vi "Ex5strip5GraphNI.vi"() -> ()   [LabVIEW 2010]
panel:
  in  "Flip":bool
  in  "Reverse":bool=TRUE
  in  "Intensifier Mode":enum16{"Safe", "Shutter", "Gate"}(ring)
  in  "IntensifierGain":u32=100
  out "Segment 5":T1(graph)
  out "Segment 4":T1(graph)
  out "Segment 3":T1(graph)
  out "Segment 2":T1(graph)
  out "Segment 1":T1(graph)
  in  "Calibration ini":path
  in  "ROI 5 Y2":u32=240
  in  "ROI 5 Y1":u32=208
  in  "ROI 4 Y2":u32=192
  in  "ROI 4 Y1":u32=160
  in  "ROI 3 Y2":u32=144
  in  "ROI 3 Y1":u32=112
  in  "ROI 2 Y2":u32=96
  in  "ROI 2 Y1":u32=64
  in  "ROI 1 Y2":u32=48
  in  "ROI 1 Y1":u32=16
  in  "Temperature":dbl=-10.0 format="%.2f"
  in  "Exposure":dbl=0.1 min=0.0 step=0.001 format="%.3f"
  in  "stop":bool
  out "error out":errorcluster
  in  "error in (no error)":errorcluster
  # "Calibration ini file"
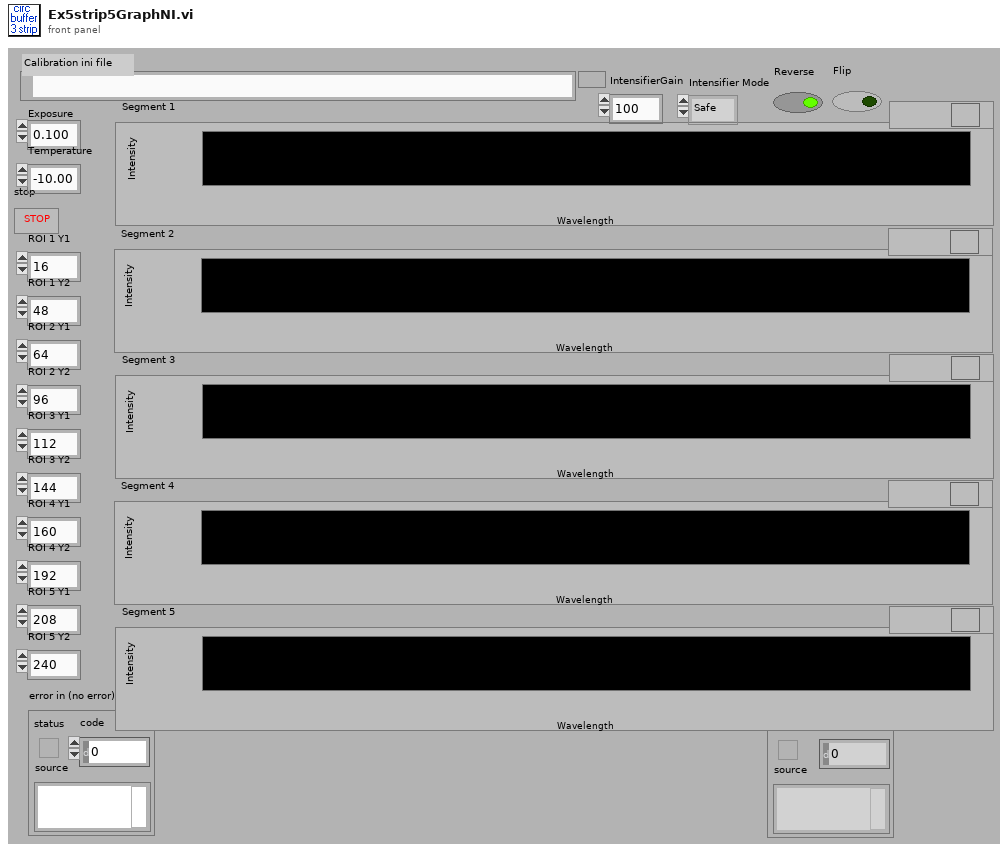
[diagram p1: front panel]
types:
  T1 = cluster{"Calibrated Array":dbl[], "Array F32":sgl[]}
  T2 = cluster{"ROI 1 Y1":u32, "ROI 1 Y2":u32, "ROI 2 Y1":u32, "ROI 2 Y2":u32, "ROI 3 Y1":u32, "ROI 3 Y2":u32, "ROI 4 Y1":u32, "ROI 4 Y2":u32, "ROI 5 Y1":u32, "ROI 5 Y2":u32}
  T3 = cluster{"Acquire focus mode,\nSync (circualar buffers)":i32, "Exposure":dbl, "Number of Images":i32, "Software Accumulation":i32}
  T4 = cluster{"Camera Handle":u32, "Pulser Handle":u32, "File Handle":u32, "Display Handle":u32, "Image Handle":u32}
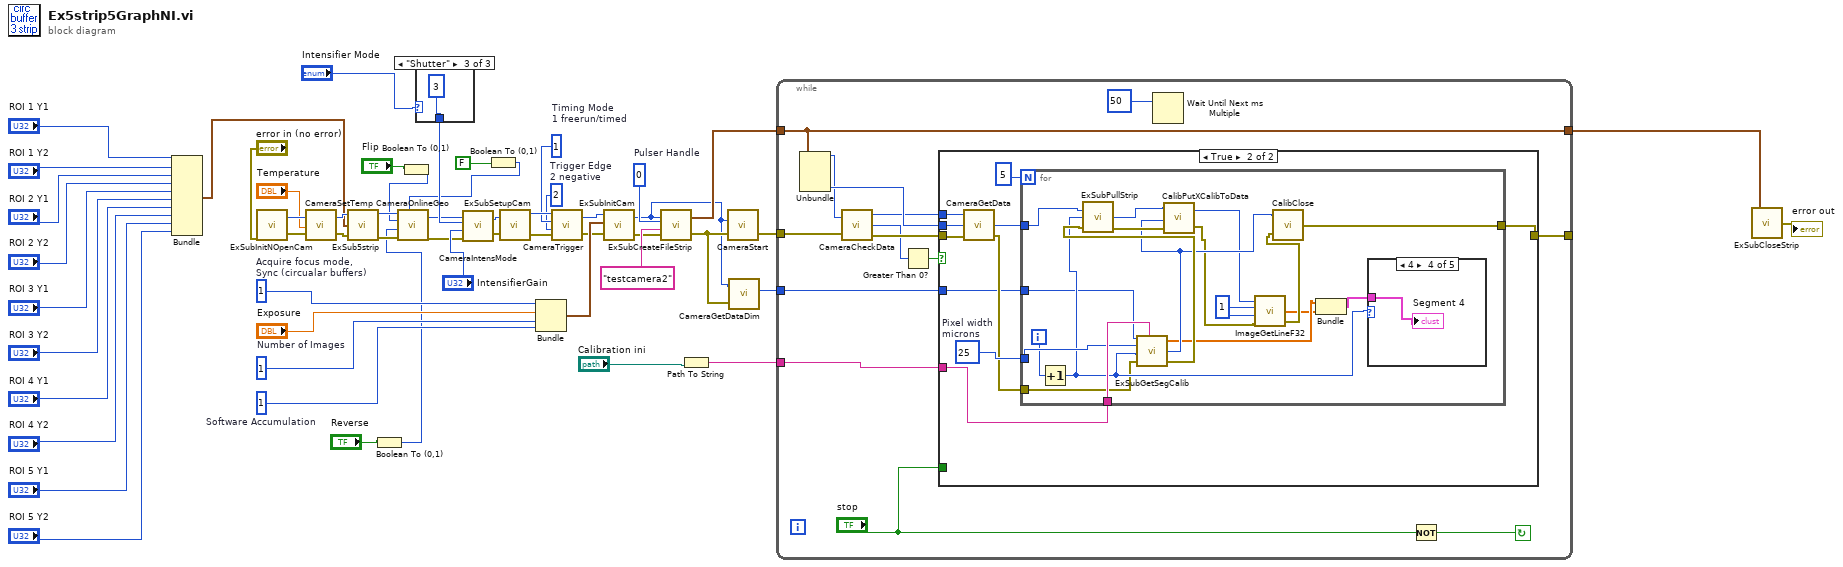
[diagram p0: block diagram]
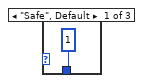
[diagram p2: hidden frame]
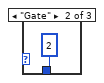
[diagram p3: hidden frame]
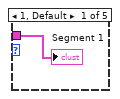
[diagram p5: hidden frame]
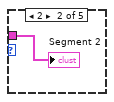
[diagram p6: hidden frame]
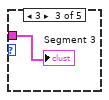
[diagram p7: hidden frame]
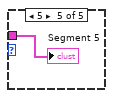
[diagram p8: hidden frame]
diagram:
  w39 = 2  # Trigger Edge 2 negative
  w40 = 1  # Timing Mode 1 freerun/timed
  w47 = 0  # Pulser Handle
  w53 = 1  # Number of Images
  w54 = 1  # Acquire focus mode, Sync (circualar buffers)
  w52 = 1  # Software Accumulation
  n1 = Bundle("ROI 1 Y1"="ROI 1 Y1", "ROI 1 Y2"="ROI 1 Y2", "ROI 2 Y1"="ROI 2 Y1", "ROI 2 Y2"="ROI 2 Y2", "ROI 3 Y1"="ROI 3 Y1", "ROI 3 Y2"="ROI 3 Y2", "ROI 4 Y1"="ROI 4 Y1", "ROI 4 Y2"="ROI 4 Y2", "ROI 5 Y1"="ROI 5 Y1", "ROI 5 Y2"="ROI 5 Y2") -> (w21:T2)  [unwired: 1 in]
  n2 = call "ExSubInitNOpenCam.vi"("error in (no error)"="error in (no error)") -> ("Camera Handle"=w34:u32, "error out"=w35:errorcluster)
  n3 = call <userlib>:"CameraSetTemp.vi"("error in (no error)"=w35, "Temperature"="Temperature", "Camera Handle"=w34) -> ("error out"=w36:errorcluster, "Camera Handle"=w33:u32)
  n4 = call "ExSub5strip.vi"("error in (no error)"=w36, "5 ROIS"=w21, "Camera Handle"=w33) -> ("error out"=w8:errorcluster, "Camera Handle"=w7:u32)
  n5 = Boolean To (0,1)(Boolean="Reverse") -> (0, 1=w3:i16)
  n6 = Boolean To (0,1)(Boolean="Flip") -> (0, 1=w5:i16)
  n7 = case shown="\"Shutter\"" "Intensifier Mode" {
    tunnel: [1 2 3] -> w15
    frame "Safe", Default {
    }
    frame "Gate" {
    }
    frame "Shutter" {
    }
  }
  n8 = Boolean To (0,1)(Boolean=FALSE) -> (0, 1=w1:i16)
  n9 = call <userlib>:"CameraOnlineGeo.vi"("Camera Handle"=w7, "Flip Flag"=w5, "Reverse Flag"=w3, "error in"=w8, "Rotate Flag"=w1) -> ("Camera Handle"=w10:u32, "error out"=w9:errorcluster)
  n10 = call <userlib>:"CameraIntensMode.vi"("error in"=w9, "Intensifier Gain"="IntensifierGain", "Mode"=w15, "Camera Handle"=w10) -> ("error out"=w14:errorcluster, "Camera Handle"=w13:u32)
  n11 = call "ExSubSetupCam.vi"("error in (no error)"=w14, "Camera Handle"=w13) -> ("error out"=w38:errorcluster, "Camera Handle"=w42:u32)
  n12 = Bundle("Acquire focus mode,\nSync (circualar buffers)"=w54, "Exposure"="Exposure", "Number of Images"=w53, "Software Accumulation"=w52) -> (w49:T3)  [unwired: 1 in]
  n13 = call <userlib>:"CameraTrigger.vi"("error in"=w38, "Trigger Edge"=w39, "Timing Mode"=w40, "Camera Handle"=w42) -> ("error out"=w43:errorcluster, "Camera Handle"=w41:u32)
  n14 = call "ExSubInitCam.vi"("error in (no error)"=w43, "Camera Information"=w49, "Camera Handle"=w41) -> ("error out"=w48:errorcluster, "Camera Handle"=w17:u32)
  n15 = call "ExSubCreateFileStrip.vi"("error in (no error)"=w48, "File and Display Name"="testcamera2", "Pulser Handle"=w47, "Camera Handle"=w17) -> ("error out"=w18:errorcluster, "Handles Out"=w46:T4)
  n16 = Path To String(path="Calibration ini") -> (string=w19:string)
  n17 = call <userlib>:"CameraStart.vi"("error in"=w18, "Camera Handle"=w17) -> ("error out"=w37:errorcluster)  [unwired: 1 out]
  n18 = call <userlib>:"CameraGetDataDim.vi"("Camera Handle"=w17, "error in"=w18) -> ("Xdim"=w16:u32)  [unwired: 3 out]
  n19 = while {
    tunnel: w46 -> [w70]
    tunnel: w37 -> [w69]
    tunnel: [w67] -> _
    tunnel: [w70] -> w45
    tunnel: w19 -> [w61]
    tunnel: w16 -> [w59]
    stop <- w71 continue-if-true
    n20 = Unbundle(w70) -> ("Camera Handle"=w65:u32, "Image Handle"=w66:u32)  [unwired: 3 out]
    n21 = call <userlib>:"CameraCheckData.vi"("Camera Handle"=w65, "error in"=w69) -> ("Camera Handle"=w64:u32, "Number Of Frames Available"=w62:i32, "error out"=w68:errorcluster)
    n22 = Greater Than 0?(x=w62) -> (x > 0?=w63:bool)
    n23 = case shown="True" w63 {
      tunnel: w68 -> [w73 w83]
      tunnel: [w73 w76] -> w67
      tunnel: w66 -> [_ w82]
      tunnel: w64 -> [_ w81]
      tunnel: w61 -> [_ w78]
      tunnel: "stop" -> [_ _]
      tunnel: w59 -> [_ w74]
      frame False {
      }
      frame True {
        w79 = 25  # Pixel width microns
        n24 = call <userlib>:"CameraGetData.vi"("error in"=w83, "Data Handle"=w82, "Camera Handle"=w81) -> ("error out"=w75:errorcluster, "Data Handle"=w77:u32)  [unwired: 1 out]
        n25 = for {
          N: 5 -> [_]
          tunnel: w78 -> [w102]
          tunnel: w79 -> [w101]
          tunnel: w77 -> [w95]
          tunnel: [w90] -> w76
          tunnel: w75 -> [w87]
          tunnel: w74 -> [w86]
          i -> [w100]
          w88 = 1
          n26 = Increment(x=w100) -> (x+1=w94:i32)
          n27 = call "ExSubGetSegCalib.vi"("x dimension"=w86, "Pixel width"=w101, "Segment number"=w94, "error in (no error)"=w87, "ini file"=w102) -> ("Calibrated Array"=w85:dbl[], "Calibration Handle"=w96:u32, "error out"=w99:errorcluster)
          n28 = call "ExSubPullStrip.vi"("error in (no error)"=w99, "Strip to pull out"=w94, "Image Handle"=w95) -> ("error out"=w98:errorcluster, "New Image Handle"=w97:u32)  [unwired: 1 out]
          n29 = call <userlib>:"CalibPutXCalibToData.vi"("error in (no error)"=w98, "Calibration Handle"=w96, "Data Handle"=w97) -> ("error out"=w92:errorcluster, "Data Handle"=w89:u32)
          n30 = call <userlib>:"ImageGetLineF32.vi"("error in"=w92, "Z Position"=w88, "Y Position"=w88, "Data Handle"=w89) -> ("error out"=w91:errorcluster, "Array F32"=w84:sgl[])  [unwired: 1 out]
          n31 = call <userlib>:"CalibClose.vi"("error in"=w91, "Calibration Handle"=w96) -> ("error out"=w90:errorcluster)
          n32 = Bundle("Calibrated Array"=w85, "Array F32"=w84) -> (w93:T1)  [unwired: 1 in]
          n33 = case shown="4" w94 {
            tunnel: w93 -> [w103 w104 w105 w106 w107]
            frame 1, Default {
              "Segment 1" <- w103
            }
            frame 2 {
              "Segment 2" <- w104
            }
            frame 3 {
              "Segment 3" <- w105
            }
            frame 4 {
              "Segment 4" <- w106
            }
            frame 5 {
              "Segment 5" <- w107
            }
          }
        }
      }
    }
    n34 = Wait Until Next ms Multiple(millisecond multiple=50) -> ()  [unwired: 1 out]
    n35 = Not(x="stop") -> (.not. x?=w71:bool)
  }
  n36 = call "ExSubCloseStrip.vi"("Handles In"=w45) -> ("error out"=→"error out":errorcluster)  [unwired: 1 in]
